vi "DisableControls.vi"(8 "error in (no error)":errorcluster caption="エラー入力（エラーなし）", 9 "Mode":enum16{"Enable", "Disable", "D&G"}(ring), 10 "ctl refs":refnum<vi>[](array[refnum]), 11 "ctl names":string[](array[string])) -> (0 "error out":errorcluster caption="エラー出力")   [LabVIEW 2015]
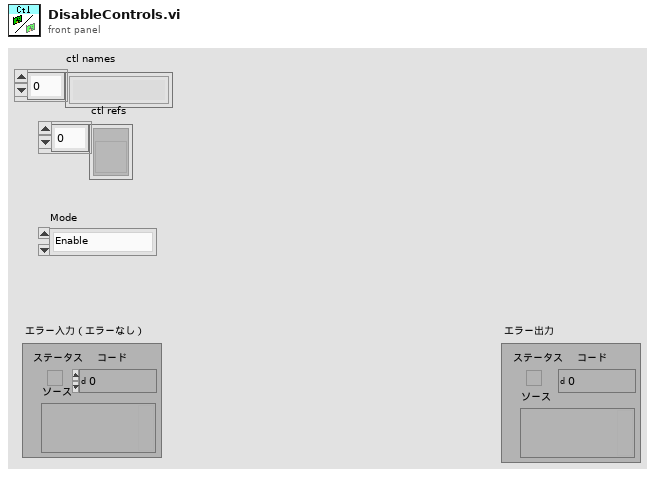
[diagram p1: front panel]
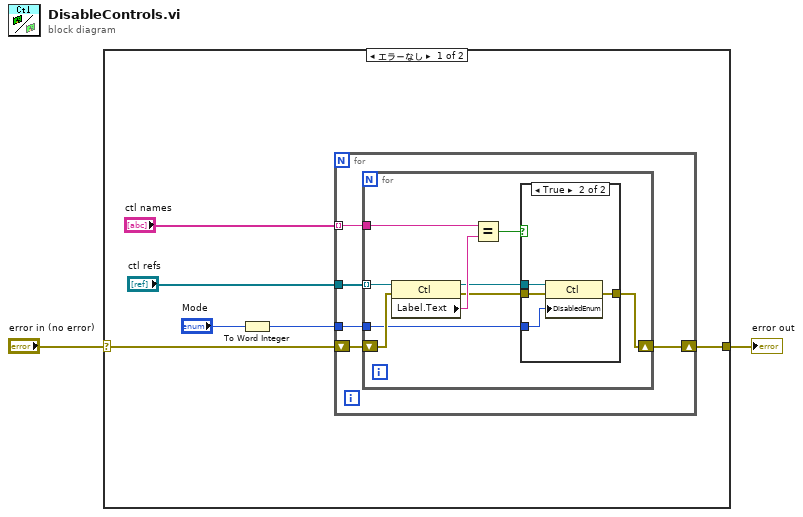
[diagram p0: block diagram]
diagram:
  n1 = case shown="エラーなし" "error in (no error)" {
    selector: "error in (no error)" -> [w6 w28]
    tunnel: [w5 w28] -> w1
    frame No Error {
      n2 = To Word Integer(number="Mode") -> (16bit integer=w3:i16)
      n3 = for {
        tunnel: "ctl names" -> [w13] mode=indexing
        tunnel: "ctl refs" -> [w12]
        shift-right: [w10] -> w5
        shift-left: w6 -> [w11]
        tunnel: w3 -> [w9]
        n4 = for {
          tunnel: w13 -> [w21]
          tunnel: w12 -> [w22] mode=indexing
          shift-right: [w16] -> w10
          shift-left: w11 -> [w17]
          tunnel: w9 -> [w14]
          n5 = property class="Ctl"(reference=w22, error in=w17) -> (reference out=w19:refnum<vi>, error out=w18:errorcluster, "Label.Text"=w20:string)
          n6 = Equal?(x=w21, y=w20) -> (x = y?=w15:bool)
          n7 = case shown="TRUE" w15 {
            tunnel: w19 -> [_ w27]
            tunnel: w18 -> [w23 w26]
            tunnel: [w23 w25] -> w16
            tunnel: w14 -> [_ w24]
            frame False {
            }
            frame True {
              n8 = property class="Ctl"(reference=w27, error in=w26, "DisabledEnum"=w24) -> (error out=w25:errorcluster)  [unwired: 1 out]
            }
          }
        }
      }
    }
    frame Error {
    }
  }
  "error out" <- w1
